vi "Read Link.vi"(7 "Reset? (F)":bool, 10 "Reset on End? (T)":bool=TRUE, 11 "Input":string) -> (2 "End?":bool, 3 "Full Output":string)   [LabVIEW 2022 SP3, in "VideoMux.lvlib" / "Mux.lvclass"]
uses:
  Mux.lvclass
  <vilib>/regexp/Match Regular Expression.xnode
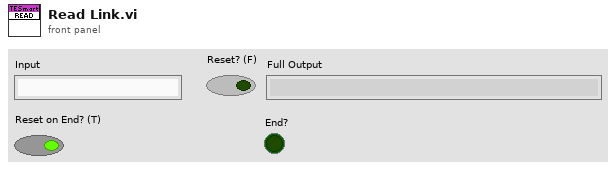
[diagram p1: front panel]
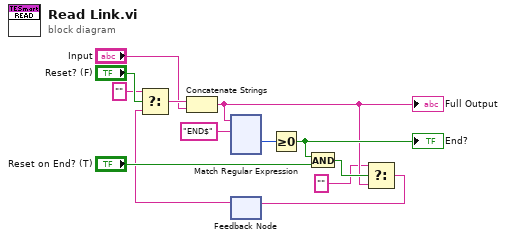
[diagram p0: block diagram]
diagram:
  n1 = feedback #1() -> (w1:string)  [unwired: 1 in]
  n2 = Select(t="", s="Reset? (F)", f=w1) -> (s? t:f=w11:string)
  n3 = Concatenate Strings(w11, "Input") -> (w4:string)
  "Full Output" <- w4
  n4 = xnode "Match Regular Expression"("input string"=w4, "regular expression"="END$") -> ("offset past match"=w8:i32)  [unwired: 4 in, 4 out]
  n5 = Greater Or Equal To 0?(x=w8) -> (x >= 0?=w6:bool)
  "End?" <- w6
  n6 = And(x=w6, y="Reset on End? (T)") -> (x .and. y?=w5:bool)
  n7 = Select(t="", s=w5, f=w4) -> (s? t:f=w2:string)
  n8 = feedback-in #1(w2) -> ()
